vi "MeasSNR.vi"(6 "IgnoreDC":bool, 7 "UpperNoiseBW":dbl=50000.0, 8 "LowerNoiseBW":dbl, 9 "VRef":dbl=1.0, 10 "FSignal":dbl=1001.0, 11 "Input":waveform(dbl)(graph)={"t0"=timestamp(0 s since 1904-01-01), "dt"=1e-05, "Y"=array[20000 elements]} caption="Histogram") -> (0 "Mag Spectrum":cluster{"f0":dbl, "df":dbl, "magnitude":dbl[]}(graph)={"f0"=0.0, "df"=5.0, "magnitude"=array[10000 elements]} caption="Histogram", 3 "MeasSNRResults":T1={"VSignalRMS"=0.7090950448868667, "VNoiseRMS"=0.09866304642333307, "SNR(dB)"=17.13099858996418, "NumBits"=2.5533220249109934, "SNRFS(dB)"=17.106609622091128, "NumBitsFS"=2.5492707013440414} {"SNRFS(dB)" format="%_3p"; "NumBitsFS" format="%.1f"; "NumBits" format="%.1f"; "SNR(dB)" format="%_3p"; "VNoiseRMS" format="%#_3p"; "VSignalRMS" format="%#_3p"})   [LabVIEW 2019]
uses:
  MeasSNRResults.ctl
  <vilib>/express/express analysis/Spectral/Block/exnSpectralBlock spectral measurements PSD poly.vi
  <vilib>/express/express analysis/Spectral/Block/exnSpectralBlock spectral measurements PSD WFM.vi
  <vilib>/express/express analysis/Spectral/Block/exnSpectralBlock spectral measurements RMS poly.vi
  <vilib>/express/express analysis/Spectral/Block/exnSpectralBlock spectral measurements RMS WFM.vi
  <vilib>/express/express analysis/Spectral/XNode/ExpressSpectralMeasurementsBlockNode.xnode
panel:
  out "SNR":dbl=7.187037807897761
  out "Input 3":dbl[](graph) caption="Histogram"
  out "input 4":dbl[](graph) caption="Histogram"
  out "PSD":cluster{"f0":dbl, "df":dbl, "magnitude":dbl[]}(graph)={"f0"=0.0, "df"=5.0, "magnitude"=array[10000 elements]} caption="Histogram"
  out "Input 2":dbl[](graph)=[1.6404078197545524e-07, 1.6087821695835617e-07, 2.2200823559551098e-07, 4.7070690663187473e-07, 8.815411911351503e-06, 0.0003227902061732271, 0.0042418373528277705, 0.020105648055654887, 0.03753178339421524, 0.02860495692959421, 0.008733116758814306, 0.0009805451787321287, 3.215521332887014e-05, 2.1451541687561014e-08, 1.966776035654292e-07, 1.41673617585858e-07, 1.3059846549443847e-07] caption="Histogram"
  out "NumBitsFS":dbl=2.5492707013440414
  out "SNRFS":dbl=17.106609622091128
  out "VSignal Max RMS":dbl=0.7071067811865475
  out "Lenght of Noise BW":dbl=10000.0
  out "Window Length":dbl=17.0
  out "starting index":dbl=192.2
  in  "Half Window Width":i32=8
  out "NumBits":dbl=2.5533220249109934
  out "SNR (dB)":dbl=17.13099858996418
  out "VNoise RMS":dbl=0.09866304642333307
  out "VSignal RMS":dbl=0.7090950448868667
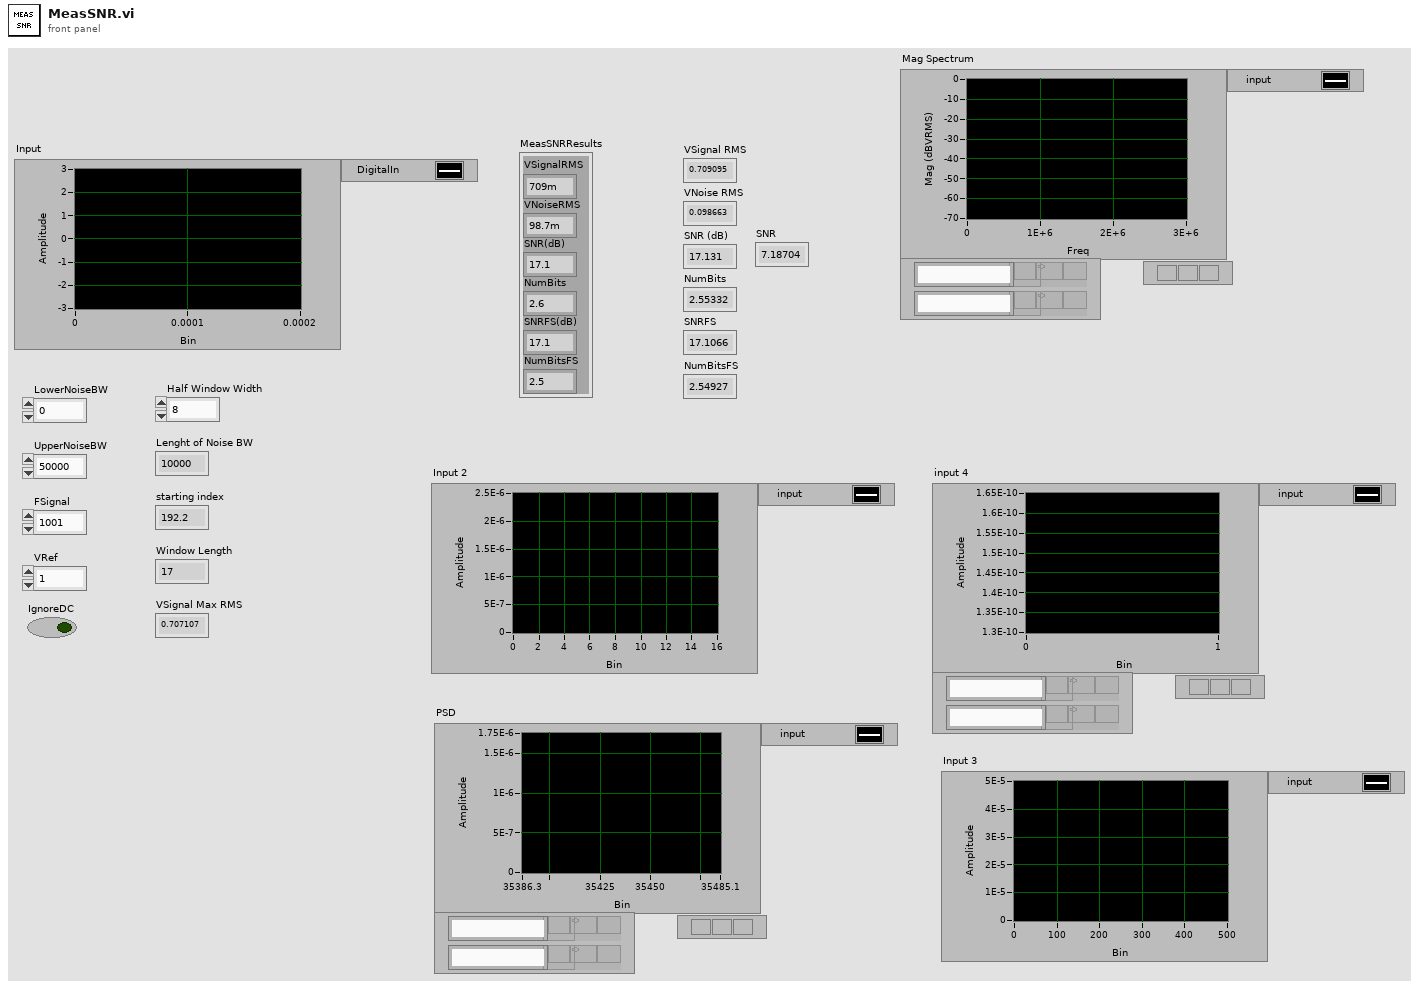
[diagram p1: front panel]
types:
  T1 = typedef "MeasSNRResults.ctl" = cluster{"VSignalRMS":dbl, "VNoiseRMS":dbl, "SNR(dB)":dbl, "NumBits":dbl, "SNRFS(dB)":dbl, "NumBitsFS":dbl}
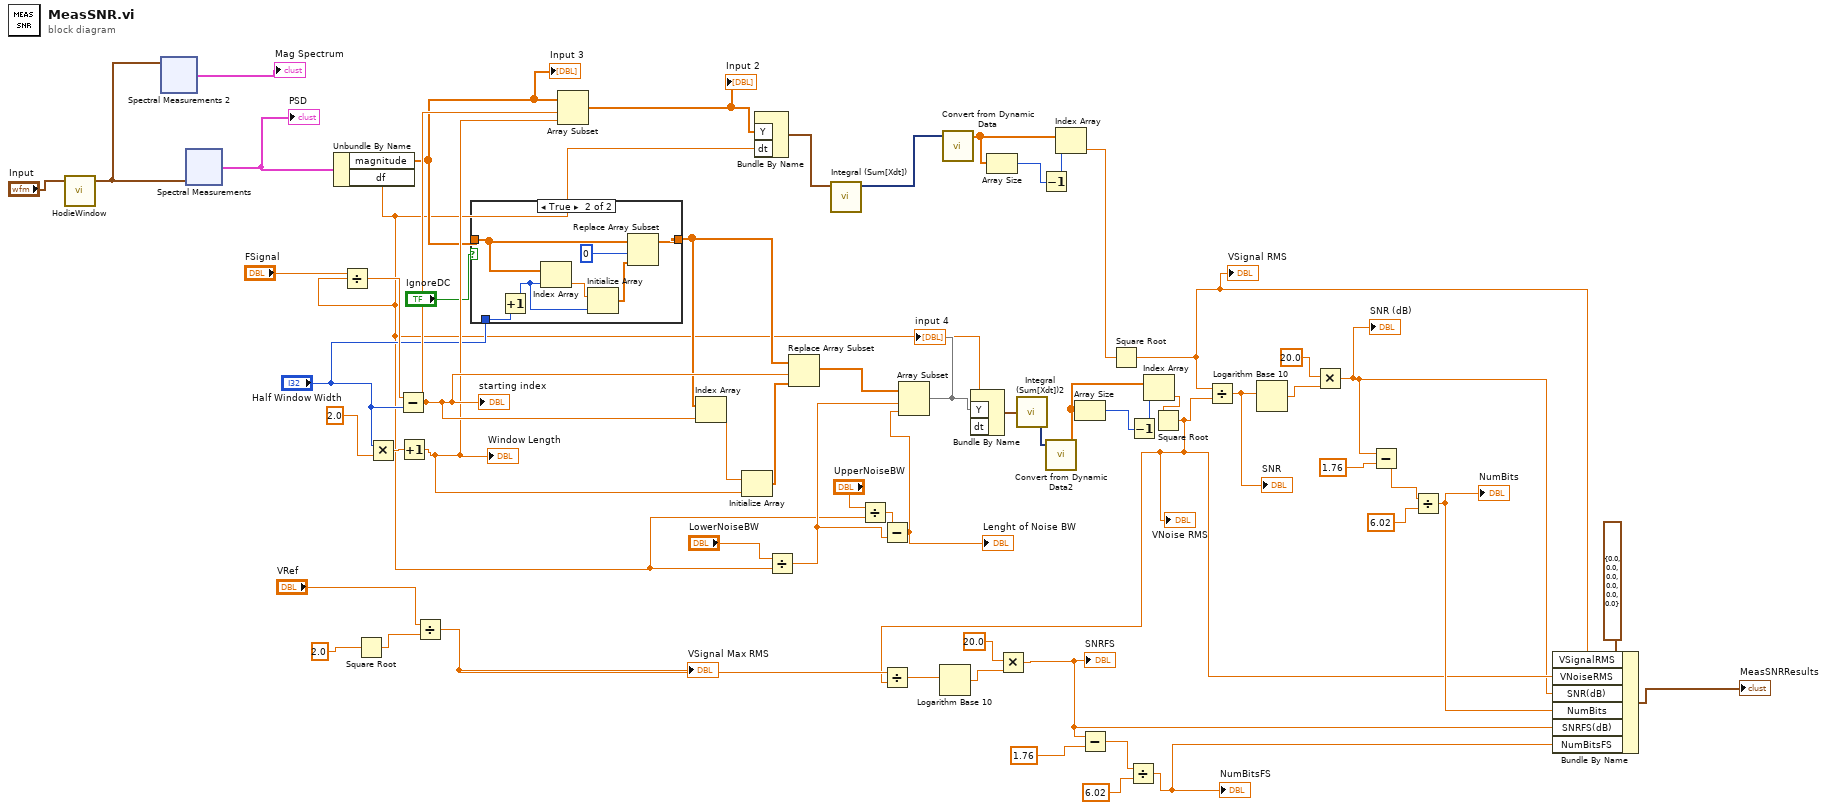
[diagram p0: block diagram]
diagram:
  n1 = call "HodieWindow.vi"("Input"="Input") -> ("Output"=w3:waveform(dbl))  [unwired: 4 in]
  n2 = xnode "Spectral Measurements 2"("Signals"=w3) -> ("FFT - (RMS)"=→"Mag Spectrum":cluster{"f0":dbl, "df":dbl, "magnitude":dbl[]})  [unwired: 1 in, 2 out]
  n3 = xnode "Spectral Measurements"("Signals"=w3) -> ("PSD"=w32:cluster{"f0":dbl, "df":dbl, "magnitude":dbl[]})  [unwired: 1 in, 1 out]
  "PSD" <- w32
  n4 = Unbundle By Name(w32) -> ("magnitude"=w7:dbl[], "df"=w1:dbl)
  "Input 3" <- w7
  n5 = Divide(x="FSignal", y=w1) -> (x/y=w53:dbl)
  n6 = Square Root(x=2.0) -> (sqrt(x)=w47:dbl)
  n7 = Multiply(x="Half Window Width", y=2.0) -> (x*y=w30:dbl)
  n8 = Subtract(x=w53, y="Half Window Width") -> (x-y=w29:dbl)
  "starting index" <- w29
  n9 = Increment(x=w30) -> (x+1=w27:dbl)
  "Window Length" <- w27
  n10 = Divide(x="VRef", y=w47) -> (x/y=w42:dbl)
  "VSignal Max RMS" <- w42
  n11 = case shown="True" "IgnoreDC" {
    tunnel: w7 -> [w62 w68]
    tunnel: [w62 w64] -> w6
    tunnel: "Half Window Width" -> [_ w67]
    frame False {
    }
    frame True {
      n12 = Increment(x=w67) -> (x+1=w66:i32)
      n13 = Index Array(array=w68, index=w66) -> (element=w63:dbl)
      n14 = Initialize Array(w63, w66) -> (w65:dbl[])
      n15 = Replace Array Subset(array=w68, new element=w65, index=0) -> (w64:dbl[])
    }
  }
  n16 = Array Subset(array=w7, index=w29, length=w27) -> (w33:dbl[])
  "Input 2" <- w33
  n17 = Index Array(array=w6, index=w29) -> (element=w55:dbl)
  n18 = Initialize Array(w55, w27) -> (w51:dbl[])
  n19 = Bundle By Name("Y"=w33, "dt"=w1) -> (w56:waveform(dbl))  [unwired: 1 in]
  n20 = Divide(x="LowerNoiseBW", y=w1) -> (x/y=w25:dbl)
  n21 = Replace Array Subset(array=w6, new element=w51, index=w29) -> (w28:dbl[])
  n22 = call "Integral (Sum[Xdt])"("Signals"=w56) -> ("Result"=w19:dynamicdata)  [unwired: 5 in, 1 out]
  n23 = Divide(x="UpperNoiseBW", y=w1) -> (x/y=w22:dbl)
  n24 = Subtract(x=w22, y=w25) -> (x-y=w50:dbl)
  "Lenght of Noise BW" <- w50
  n25 = Array Subset(array=w28, index=w25, length=w50) -> (w26:dbl[])
  "input 4" <- w26
  n26 = call "Convert from Dynamic Data"("Dynamic Data Type"=w19) -> ("Array"=w18:dbl[])  [unwired: 3 in]
  n27 = Bundle By Name("Y"=w26, "dt"=w1) -> (w49:waveform(dbl))  [unwired: 1 in]
  n28 = Array Size(array=w18) -> (size(s)=w17:i32)
  n29 = call "Integral (Sum[Xdt])2"("Signals"=w49) -> ("Result"=w11:dynamicdata)  [unwired: 5 in, 1 out]
  n30 = Decrement(x=w17) -> (x-1=w16:i32)
  n31 = call "Convert from Dynamic Data2"("Dynamic Data Type"=w11) -> ("Array"=w12:dbl[])  [unwired: 3 in]
  n32 = Index Array(array=w18, index=w16) -> (element=w15:dbl)
  n33 = Array Size(array=w12) -> (size(s)=w13:i32)
  n34 = Square Root(x=w15) -> (sqrt(x)=w21:dbl)
  "VSignal RMS" <- w21
  n35 = Decrement(x=w13) -> (x-1=w14:i32)
  n36 = Index Array(array=w12, index=w14) -> (element=w10:dbl)
  n37 = Square Root(x=w10) -> (sqrt(x)=w20:dbl)
  "VNoise RMS" <- w20
  n38 = Divide(x=w42, y=w20) -> (x/y=w44:dbl)
  n39 = Logarithm Base 10(1:w44) -> (0:w45:dbl)
  n40 = Multiply(x=20.0, y=w45) -> (x*y=w35:dbl)
  "SNRFS" <- w35
  n41 = Subtract(x=w35, y=1.76) -> (x-y=w40:dbl)
  n42 = Divide(x=w40, y=6.02) -> (x/y=w34:dbl)
  "NumBitsFS" <- w34
  n43 = Divide(x=w21, y=w20) -> (x/y=w9:dbl)
  "SNR" <- w9
  n44 = Logarithm Base 10(1:w9) -> (0:w60:dbl)
  n45 = Multiply(x=20.0, y=w60) -> (x*y=w8:dbl)
  "SNR (dB)" <- w8
  n46 = Subtract(x=w8, y=1.76) -> (x-y=w58:dbl)
  n47 = Divide(x=w58, y=6.02) -> (x/y=w36:dbl)
  "NumBits" <- w36
  n48 = Bundle By Name(cluster=T1 {"VSignalRMS"=0.0, "VNoiseRMS"=0.0, "SNR(dB)"=0.0, "NumBits"=0.0, "SNRFS(dB)"=0.0, "NumBitsFS"=0.0} ("MeasSNRResults"), "VSignalRMS"=w21, "VNoiseRMS"=w20, "SNR(dB)"=w8, "NumBits"=w36, "SNRFS(dB)"=w35, "NumBitsFS"=w34) -> (→"MeasSNRResults":T1)
